vi "Play Selector.vi"() -> (0 "Output Play":T1)   [LabVIEW 2016]
uses:
  Autonomous Play Definition.ctl
  Autonomous Commands/Autonomous Command Names.ctl
  <vilib>/Rock Robotics/Network Tables/SD Read String.vi
  Global Variables/File Path Globals.vi
  Global Variables/Autonomous Exec Info.vi
panel:
  out "error out":errorcluster
  out "rest of the binary string":string
  out "File Name of Play":string
  # "Add as many plays \nas needed or are supported\nby the number of bits in\nplay selector\n\nRemember Ryan wants \nno less than 32 \nautonomous plays\n\nREMEMBER TO SAVE ALL \nVALUES AS DEFAULT \nEVERYTIME YOU MAKE \nCHANGES TO PLAYS"
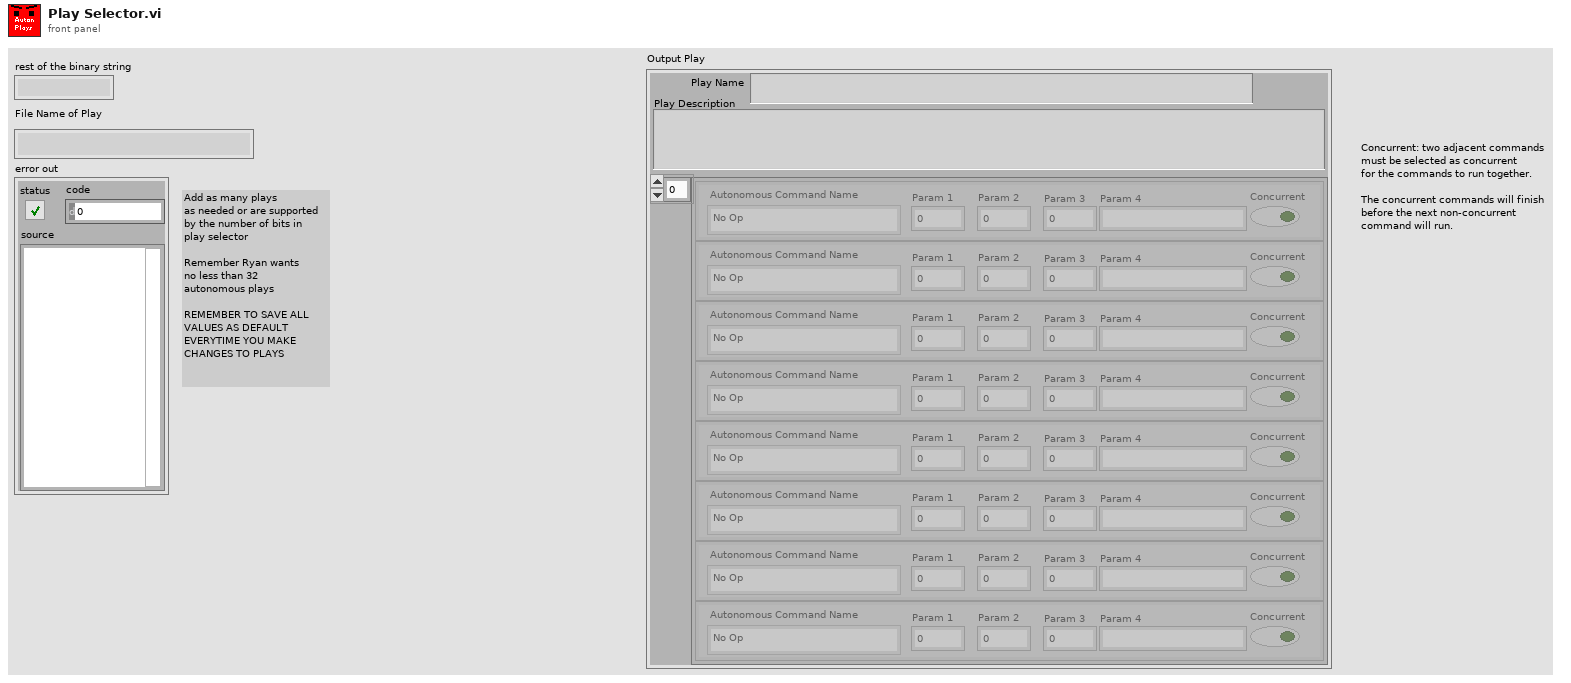
[diagram p1: front panel]
types:
  T1 = typedef "Autonomous Play Definition.ctl" = cluster{"Play Name":string, "Command List":cluster{"Param 1":dbl, "Param 2":dbl, "Autonomous Command Name":T2, "Concurrent":bool, "Param 3":dbl, "Param 4":string}[], "Play Description":string}
  T2 = typedef "Autonomous Command Names.ctl" = enum16{"No Op", "Command Drive+Climb Shift", "Command Wait", "Command Deliver Gear", "Command Buffer", "Command Drive Path", "Command Drive Time", "Command Shoot", "Command Turn to Heading", "Command Run Conveyor", "Command Spinup Shooter", "Command Deliver Gear Front", "Command Toggle Intake Rotation", "DO NOT USE", "Command Agitate Hopper", "Command Pre-Buffer", "Command Turn to Target", "Command Deliver Gear with Safety", "Command Drive Time with IMU", "Command Drive to Encoders"}
  T3 = cluster{"Param 1":dbl, "Param 2":dbl, "Autonomous Command Name":T2, "Concurrent":bool, "Param 3":dbl, "Param 4":string}[]
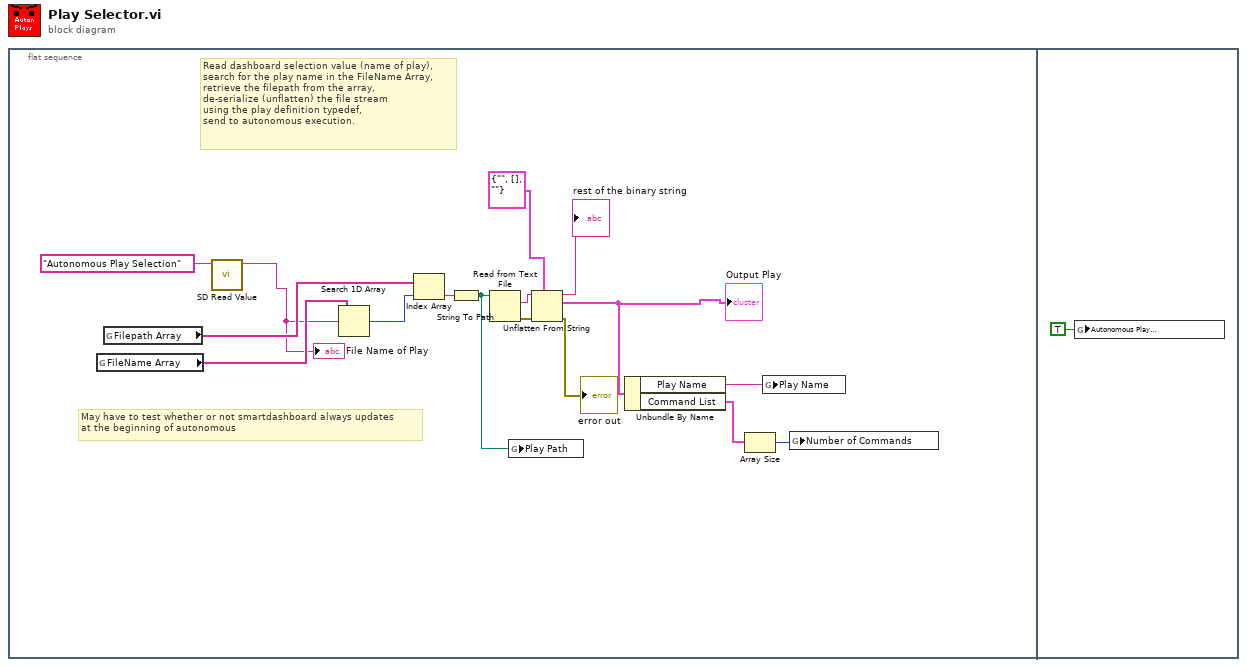
[diagram p0: block diagram]
diagram:
  n1 = flat-sequence {
    frame #0 {
      # "May have to test whether or not smartdashboard always updates\nat the beginning of autonomous"
      # "Read dashboard selection value (name of play), \nsearch for the play name in the FileName Array,\nretrieve the filepath from the array,\nde-serialize (unflatten) the file stream\nusing the play definition typedef, \nsend to autonomous execution."
      n2 = global read "File Path Globals.vi" "FileName Array"() -> (w16:string[])
      n3 = global read "File Path Globals.vi" "Filepath Array"() -> (w15:string[])
      n4 = call-poly <vilib>:"SD Read Value.vi"("Name"="Autonomous Play Selection") -> ("String"=w2:string)  [unwired: 8 in, 2 out]
      "File Name of Play" <- w2
      n5 = Search 1D Array(1D array=w16, element=w2) -> (index of element=w14:i32)  [unwired: 1 in]
      n6 = Index Array(array=w15, index=w14) -> (element=w13:string)
      n7 = String To Path(string=w13) -> (path=w5:path)
      n8 = Read from Text File(file (use dialog)=w5) -> (text=w12:string, error out=w9:errorcluster)  [unwired: 3 in, 2 out]
      n9 = global write "Autonomous Exec Info.vi" "Play Path"(w5) -> ()
      n10 = Unflatten From String(type=T1 {"Play Name"="", "Command List"=[], "Play Description"=""}, binary string=w12, error in (no error)=w9) -> (rest of the binary string=→"rest of the binary string":string, value=w3:T1, error out=→"error out":errorcluster)  [unwired: 2 in]
      "Output Play" <- w3
      n11 = Unbundle By Name(w3) -> ("Play Name"=w8:string, "Command List"=w7:T3)
      n12 = Array Size(array=w7) -> (size(s)=w6:i32)
      n13 = global write "Autonomous Exec Info.vi" "Play Name"(w8) -> ()
      n14 = global write "Autonomous Exec Info.vi" "Number of Commands"(w6) -> ()
    }
    frame #1 {
      n15 = global write "Autonomous Exec Info.vi" "Autonomous Play\nRead"(TRUE ("Autonomous Play\nRead")) -> ()
    }
  }
